vi "Launcher.vi"() -> ()   [LabVIEW 2020]
uses:
  GUI Generador/GUI Generador.lvclass
  <vilib>/ActorFramework/Actor/Actor.lvclass
  C:/Program Files (x86)/National Instruments/LabVIEW 2020/vi.lib/ActorFramework/Actor/Actor.lvclass
panel:
  in  "Stop":bool
  in  "Sentencia un actor":enum16{""}(ring)
  in  "Matar":bool
  in  "Actores":enum16{"Binario", "Generador"}(ring)
  in  "Nuevo":bool
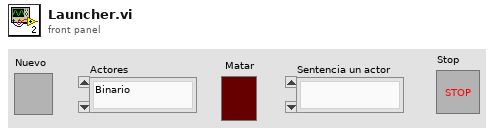
[diagram p1: front panel]
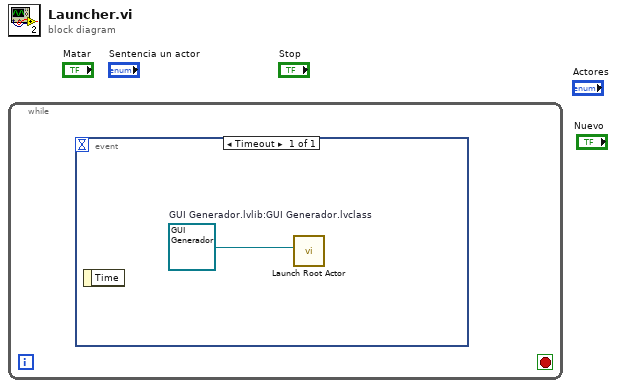
[diagram p0: block diagram]
diagram:
  n1 = while {
    stop <- _ stop-if-true
    n2 = event shown="[0] Timeout" {
      selector: _ -> [_]
      dyn-events: _ -> [_]
      timeout: _ -> [_]
      event Timeout {
        w1 = refnum<class "GUI Generador.lvclass"> refnum  # GUI Generador.lvlib:GUI Generador.lvclass
        n3 = event-data() -> ()  [unwired: 1 in, 1 out]
        n4 = call <vilib>:"Launch Root Actor.vi"("Actor"=w1) -> ()  [unwired: 9 in, 2 out]
      }
    }
  }
